vi "Update JLink Command File.vi"(7 "Flash Programming Command Type":T1, 8 "error in (no error)":errorcluster, 10 "Flash Programming Configuration":T2={"Erase Configuration"={"Start Address"="", "End Address"="", "Reset"=TRUE}, "LoadFile Configuration"={"File Name"=path "", "Address"="", "Reset"=TRUE}}) -> (0 "error out":errorcluster, 2 "Command":string, 3 "J-Link Command File":path)   [LabVIEW 2016, in "JLink Commander.lvlib"]
doc: "Update J-Link Command File (.jlink) based on the Flash Programming Configuration inputs."
uses:
  JLink Commander.lvlib
  Type Definitions/Flash Programming Configuration.ctl
  Type Definitions/Flash Programming Command Type.ctl
  <vilib>/Utility/file.llb/Read Delimited Spreadsheet (string).vi
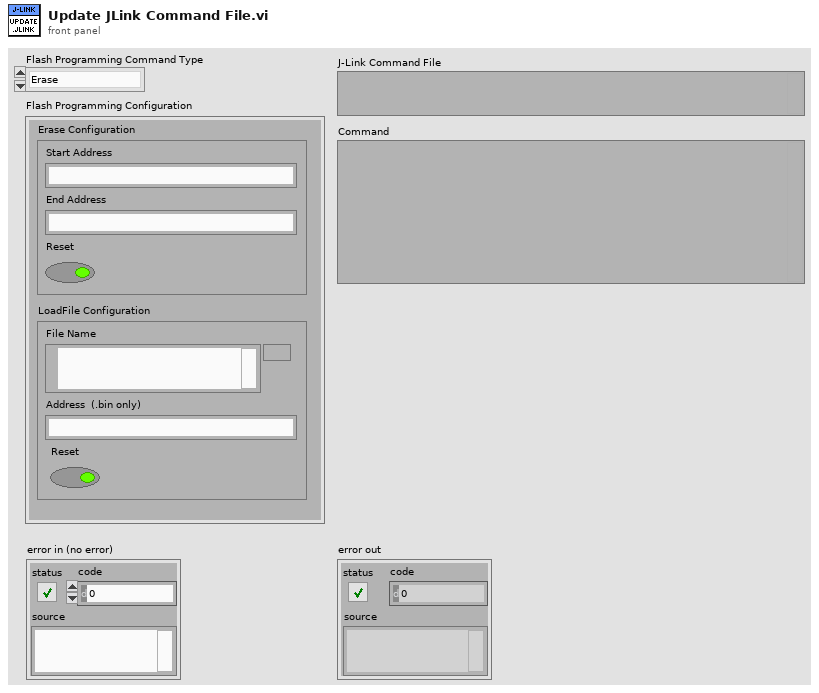
[diagram p1: front panel]
types:
  T1 = typedef "JLink Commander.lvlib/Flash Programming Command Type.ctl" = enum16{"Erase", "ReadBinary", "LoadFile", "SaveBin", "VerifyBin"}
  T2 = typedef "JLink Commander.lvlib/Flash Programming Configuration.ctl" = cluster{"Erase Configuration":cluster{"Start Address":string, "End Address":string, "Reset":bool}, "LoadFile Configuration":cluster{"File Name":path, "Address":string, "Reset":bool}}
  T3 = enum16{"open", "replace", "create", "open or create", "replace or create", "replace or create with confirmation"}
  T4 = cluster{"Start Address":string, "End Address":string, "Reset":bool}
  T5 = cluster{"File Name":path, "Address":string, "Reset":bool}
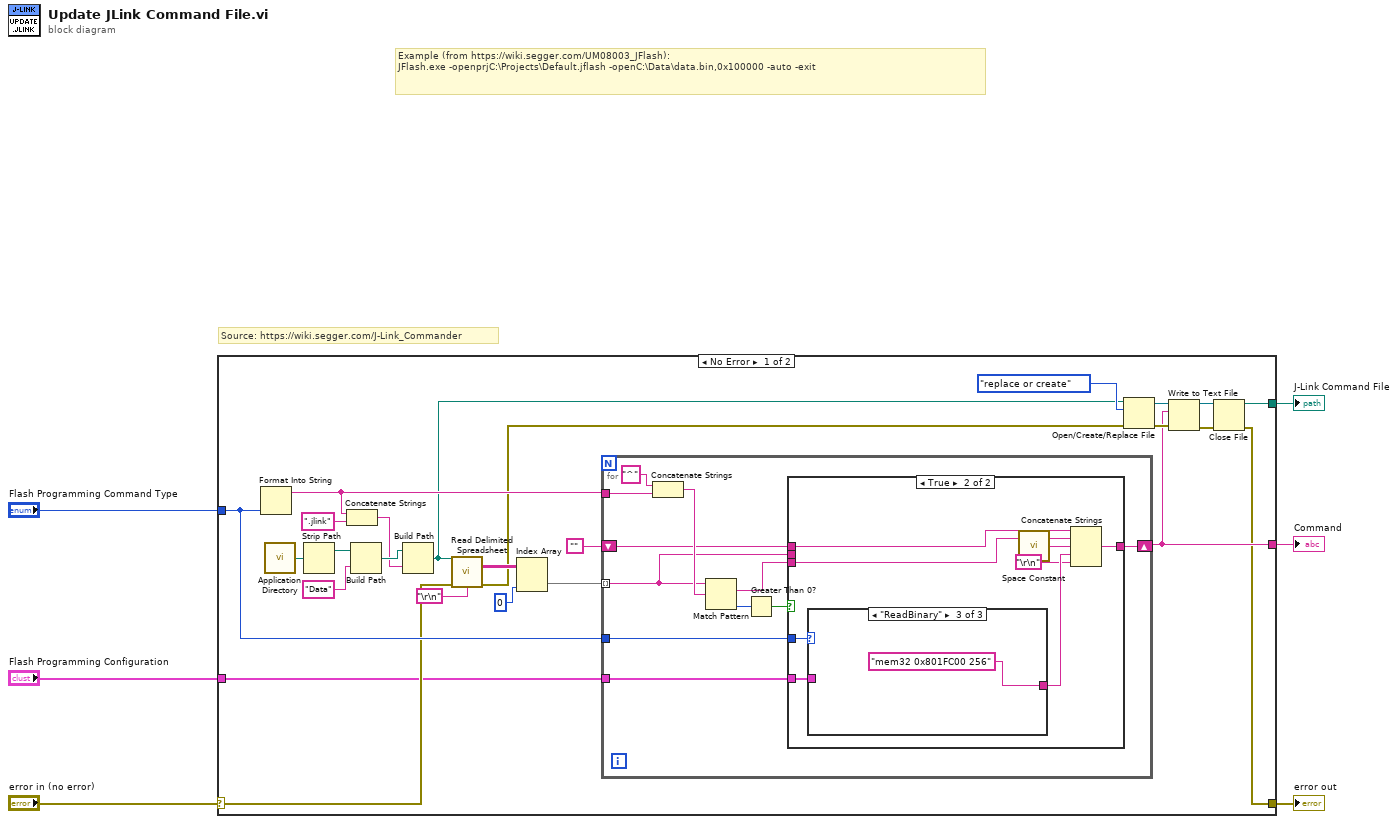
[diagram p0: block diagram]
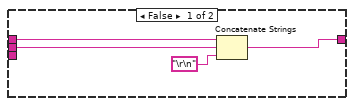
[diagram p2: hidden frame]
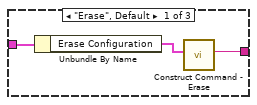
[diagram p3: hidden frame]
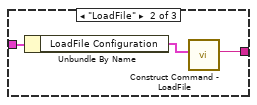
[diagram p4: hidden frame]
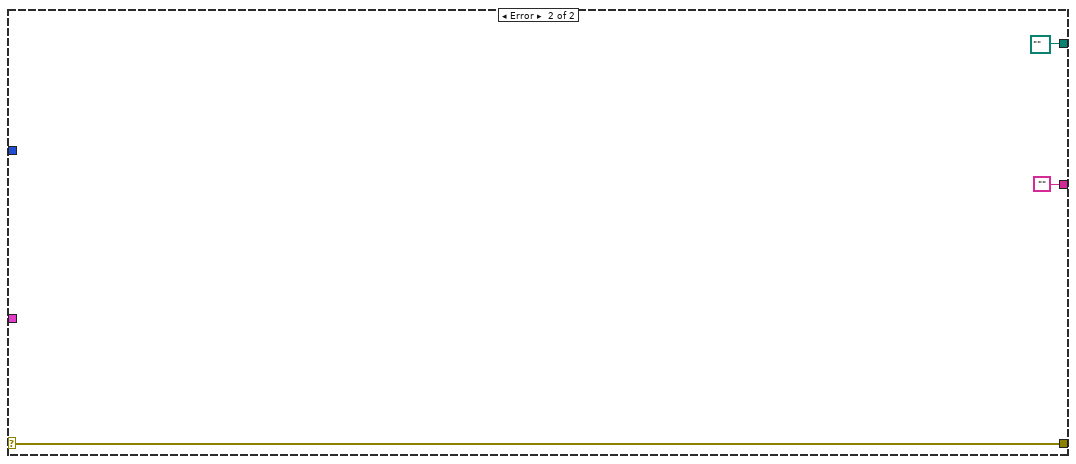
[diagram p5: hidden frame]
diagram:
  # "Source: https://wiki.segger.com/J-Link_Commander"
  # "Example (from https://wiki.segger.com/UM08003_JFlash):\nJFlash.exe -openprjC:\\Projects\\Default.jflash -openC:\\Data\\data.bin,0x100000 -auto -exit"
  n1 = case shown="No Error" "error in (no error)" {
    selector: "error in (no error)" -> [w15 w64]
    tunnel: [w17 w64] -> w5
    tunnel: "Flash Programming Command Type" -> [w24 _]
    tunnel: [w18 ""] -> w4
    tunnel: [w13 path "" ("path")] -> w3
    tunnel: "Flash Programming Configuration" -> [w12 _]
    frame No Error {
      n2 = Format Into String(w24) -> (resulting string=w27:string)  [unwired: 3 in, 1 out]
      n3 = call <vilib>:"Application Directory.vi"() -> ("Application Directory"=w11:path)
      n4 = Strip Path(path=w11) -> (stripped path=w10:path)  [unwired: 1 out]
      n5 = Concatenate Strings(w27, ".jlink" ("string")) -> (w7:string)
      n6 = Build Path(base path=w10, name or relative path="Data") -> (appended path=w9:path)
      n7 = Build Path(base path=w9, name or relative path=w7) -> (appended path=w16:path)
      n8 = call-poly <vilib>:"Read Delimited Spreadsheet.vi"("file path (dialog if empty)"=w16, "error in (no error)"=w15, "delimiter (\\t)"="\r\n" ("delimiter (\\t)")) -> ("all rows"=w30:string[][], "error out"=w14:errorcluster)  [unwired: 7 in, 4 out]
      n9 = Index Array(array=w30, index (col)=0 ("disabled index (col)")) -> (element=w28:string[])  [unwired: 1 in]
      n10 = for {
        tunnel: w28 -> [w36] mode=indexing
        tunnel: w27 -> [w41]
        shift-right: [w38] -> w18
        shift-left: "" -> [w37]
        tunnel: w24 -> [w35]
        tunnel: w12 -> [w32]
        n11 = Concatenate Strings("^" ("string"), w41) -> (w39:string)
        n12 = Match Pattern(string=w36, regular expression=w39) -> (match substring=w34:string, offset past match=w42:i32)  [unwired: 1 in, 2 out]
        n13 = Greater Than 0?(x=w42) -> (x > 0?=w33:bool)
        n14 = case shown="True" w33 {
          tunnel: [w43 w52] -> w38
          tunnel: w37 -> [w46 w48]
          tunnel: w36 -> [w44 _]
          tunnel: w35 -> [_ w54]
          tunnel: w34 -> [_ w51]
          tunnel: w32 -> [_ w47]
          frame False {
            n15 = Concatenate Strings(w46, w44, "\r\n") -> (w43:string)
          }
          frame True {
            n16 = case shown="\"ReadBinary\"" w54 {
              tunnel: [w57 w60 "mem32 0x801FC00 256" ("Command")] -> w53
              tunnel: w47 -> [w56 w59 _]
              frame "Erase", Default {
                n17 = Unbundle By Name(w56) -> ("Erase Configuration"=w55:T4)
                n18 = call "Construct Command - Erase.vi"("Erase Configuration"=w55) -> ("Command"=w57:string)  [unwired: 9 in, 1 out]
              }
              frame "LoadFile" {
                n19 = Unbundle By Name(w59) -> ("LoadFile Configuration"=w58:T5)
                n20 = call "Construct Command - LoadFile.vi"("LoadFile Configuration"=w58) -> ("Command"=w60:string)  [unwired: 9 in, 1 out]
              }
              frame "ReadBinary" {
              }
            }
            n21 = call <vilib>:"Space Constant.vi"() -> ("String"=w50:string)
            n22 = Concatenate Strings(w48, w51, w50, w53, "\r\n") -> (w52:string)
          }
        }
      }
      n23 = Open/Create/Replace File(file path (use dialog)=w16, error in=w14, operation (0:open)=T3."replace or create") -> (refnum out=w23:refnum<file>, error out=w20:errorcluster)  [unwired: 3 in, 1 out]
      n24 = Write to Text File(file (use dialog)=w23, text=w18, error in=w20) -> (refnum out=w22:refnum<file>, error out=w21:errorcluster)  [unwired: 1 in, 1 out]
      n25 = Close File(refnum=w22, error in=w21) -> (path=w13:path, error out=w17:errorcluster)
    }
    frame Error {
    }
  }
  "error out" <- w5
  "Command" <- w4
  "J-Link Command File" <- w3
